vi "Correct Offset.vi"(10 "Translation":dbl[](array[numeric]), 11 "YPR (deg)":cluster{"yaw":dbl, "pitch":dbl, "roll":dbl} {"yaw" format="%.1g"; "pitch" format="%.1g"; "roll" format="%.1g"}) -> (2 "Adjusted Translation":dbl[](array[numeric]))   [LabVIEW 2025]
panel:
  in  "scale":dbl=2.0
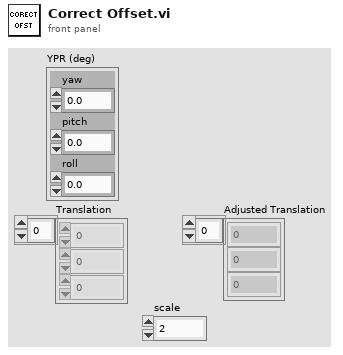
[diagram p1: front panel]
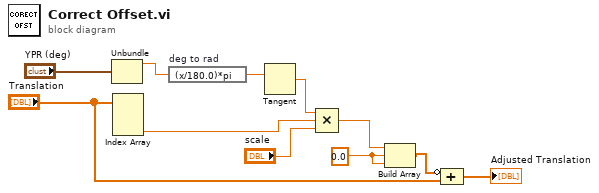
[diagram p0: block diagram]
diagram:
  w6 = 0.0
  n1 = Unbundle("YPR (deg)") -> ("yaw"=w2:dbl)  [unwired: 2 out]
  n2 = Index Array(array="Translation") -> (element #3=w10:dbl)  [unwired: 3 in, 2 out]
  n3 = expression code="(x/180.0)*pi" "deg to rad"(w2) -> (w3:dbl)
  n4 = Tangent(1:w3) -> (0:w4:dbl)
  n5 = Compound Arithmetic op=MULTIPLY(w4, w10, "scale") -> (w5:dbl)
  n6 = Build Array(w5, w6, w6) -> (w8:dbl[])
  n7 = Compound Arithmetic op=ADD(invert w8, "Translation") -> (→"Adjusted Translation":dbl[])
